vi "PWM_Motor_IR.vi"(0 "Sensorwert":dbl, 1 "Geschwindigkeit multiplikator":dbl(knob) scale=0.0..1.0) -> (6 "PWM Motor":dbl=0.3, 7 "Folgen?":bool)   [LabVIEW 2016]
doc: "Geschwindigkeitsregelung anhand IR Sensor vorne\n05.04.17_Tloe"
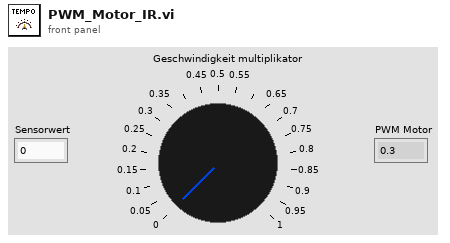
[diagram p1: front panel]
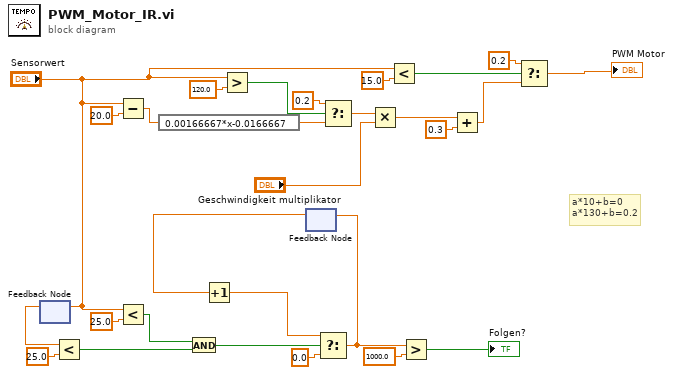
[diagram p0: block diagram]
diagram:
  # "a*10+b=0 \na*130+b=0.2"
  n1 = feedback-in #1("Sensorwert") -> ()
  n2 = feedback #1() -> (w22:dbl)  [unwired: 1 in]
  n3 = Less?(x=w22, y=25.0) -> (x < y?=w18:bool)
  n4 = Subtract(x="Sensorwert", y=20.0) -> (x-y=w9:dbl)
  n5 = Less?(x="Sensorwert", y=25.0) -> (x < y?=w19:bool)
  n6 = expression code="0.00166667*x-0.0166667"(w9) -> (w7:dbl)
  n7 = And(x=w19, y=w18) -> (x .and. y?=w17:bool)
  n8 = Greater?(x="Sensorwert", y=120.0) -> (0:w27:bool)
  n9 = feedback #2() -> (w14:dbl)  [unwired: 1 in]
  n10 = Increment(x=w14) -> (x+1=w15:dbl)
  n11 = Select(t=w15, s=w17, f=0.0) -> (s? t:f=w13:dbl)
  n12 = feedback-in #2(w13) -> ()
  n13 = Select(t=0.2, s=w27, f=w7) -> (s? t:f=w24:dbl)
  n14 = Multiply(x=w24, y="Geschwindigkeit multiplikator") -> (x*y=w25:dbl)
  n15 = Less?(x="Sensorwert", y=15.0) -> (x < y?=w4:bool)
  n16 = Greater?(x=w13, y=1000.0) -> (0:→"Folgen?":bool)
  n17 = Add(x=w25, y=0.3) -> (x+y=w6:dbl)
  n18 = Select(t=0.2, s=w4, f=w6) -> (s? t:f=→"PWM Motor":dbl)
